vi "Export.vi"(8 "error in":errorcluster, 10 "path":path, 11 "item in":T1 format="%.0x") -> (0 "error out":errorcluster, 3 "item out":T1 format="%.0x")   [LabVIEW 2020, in "Custom Device Serialization.lvlib"]
uses:
  Custom Device Serialization.lvlib
  <vilib>/NI VeriStand/Custom Device API/Custom Device Item Ref.ctl
  <vilib>/NI VeriStand/Custom Device API/Custom Device API.lvlib
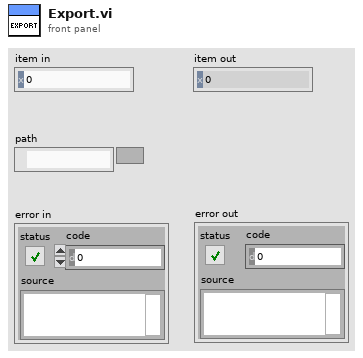
[diagram p1: front panel]
types:
  T1 = typedef "Custom Device API.lvlib/Custom Device Item Ref.ctl" = u64
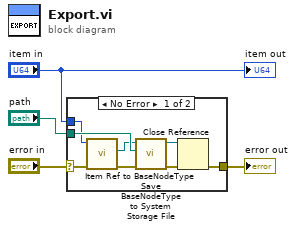
[diagram p0: block diagram]
diagram:
  n1 = case shown="No Error" "error in" {
    selector: "error in" -> [w8 w13]
    tunnel: "path" -> [w12 _]
    tunnel: [w10 w13] -> w2
    tunnel: "item in" -> [w7 _]
    frame No Error {
      n2 = call "Item Ref to BaseNodeType.vi"("error in (no error)"=w8, "item ref in"=w7) -> ("error out"=w5:errorcluster, "NationalInstruments.VeriStand.SystemStorage.BaseNodeType"=w6:refnum<k39>)  [unwired: 7 in, 1 out]
      n3 = call "Save BaseNodeType to System Storage File.vi"("error in (no error)"=w5, "path"=w12, "NationalInstruments.VeriStand.SystemStorage.BaseNodeType"=w6) -> ("error out"=w11:errorcluster, "NationalInstruments.VeriStand.SystemStorage.BaseNodeType"=w9:refnum<k39>)  [unwired: 7 in]
      n4 = Close Reference(reference=w9, error in (no error)=w11) -> (error out=w10:errorcluster)
    }
    frame Error {
    }
  }
  "error out" <- w2
  "item out" <- "item in"
